vi "Alter Macro V2.vi"(7 "Action":enum16{"Add", "Insert", "Modify", "Delete"}(ring)=enum."Delete", 9 "Step":i32, 10 "Steps in":T1[](array[typedef])) -> (2 "Steps out":T1[](array[typedef]))   [LabVIEW 2023]
doc: "Higher level VI for performing a number of actions on a profile. Takes <B>Action</B> as an input and executes code that performs that action.\n\nThis V2 is meant to be used in conjunction with the double click functionality that was put in as a patch."
uses:
  CTLs/Step Type V3.ctl
  CTLs/Step V3.ctl
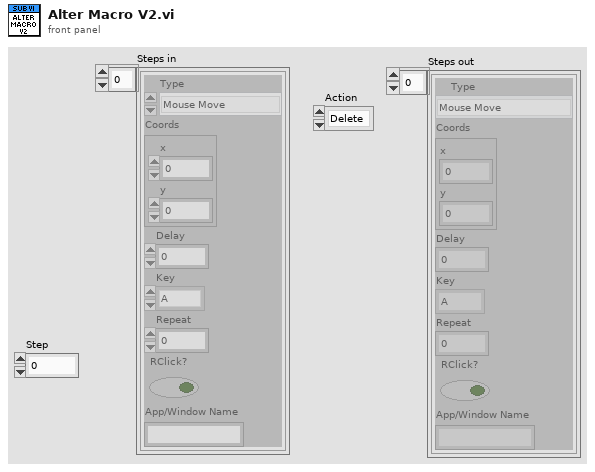
[diagram p1: front panel]
types:
  T1 = typedef "Step V3.ctl" = cluster{"Type":T2, "Coords":cluster{"x":i32, "y":i32}, "Delay":i32, "Key":u8, "Repeat":i32, "RClick?":bool, "App/Window Name":string}
  T2 = typedef "Step Type V3.ctl" = enum16{"Mouse Move", "Mouse Click", "Key Press", "Wait", "Mouse Down", "Mouse Up", "Key Down", "Key Up", "Run Application", "Quit Application", "Maximize Window", "Minimize Window", "Bring Window to Front", "Send Window to Back"}
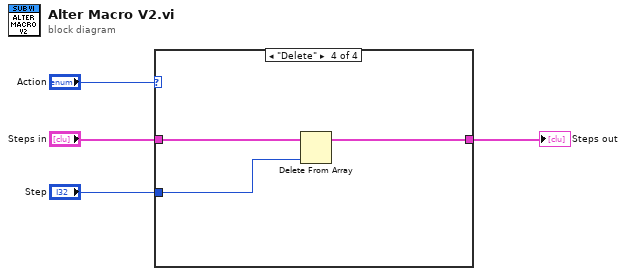
[diagram p0: block diagram]
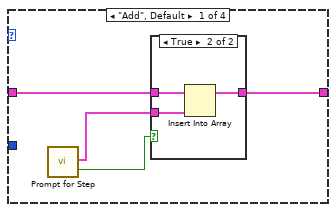
[diagram p2: hidden frame]
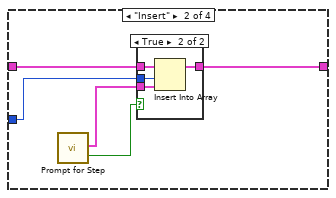
[diagram p4: hidden frame]
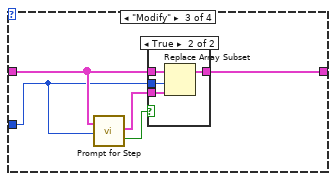
[diagram p6: hidden frame]
diagram:
  n1 = case shown="\"Delete\"" "Action" {
    tunnel: "Steps in" -> [w7 w17 w27 w35]
    tunnel: [w6 w16 w26 w34] -> w1
    tunnel: "Step" -> [_ w13 w23 w33]
    frame "Add", Default {
      n2 = call "Prompt for Step.vi"() -> ("New Data Out"=w8:T1, "OK?"=w5:bool)  [unwired: 17 in, 1 out]
      n3 = case shown="True" w5 {
        tunnel: w8 -> [_ w12]
        tunnel: w7 -> [w9 w11]
        tunnel: [w9 w10] -> w6
        frame False {
        }
        frame True {
          n4 = Insert Into Array(array=w11, new element=w12) -> (w10:T1[])  [unwired: 1 in]
        }
      }
    }
    frame "Insert" {
      n5 = call "Prompt for Step.vi"() -> ("New Data Out"=w15:T1, "OK?"=w14:bool)  [unwired: 17 in, 1 out]
      n6 = case shown="True" w14 {
        tunnel: w13 -> [_ w22]
        tunnel: w15 -> [_ w21]
        tunnel: w17 -> [w18 w20]
        tunnel: [w18 w19] -> w16
        frame False {
        }
        frame True {
          n7 = Insert Into Array(array=w20, index=w22, new element=w21) -> (w19:T1[])
        }
      }
    }
    frame "Modify" {
      n8 = call "Prompt for Step.vi"("Steps"=w27, "Index"=w23) -> ("New Data Out"=w25:T1, "OK?"=w24:bool)  [unwired: 15 in, 1 out]
      n9 = case shown="True" w24 {
        tunnel: w23 -> [_ w32]
        tunnel: w25 -> [_ w31]
        tunnel: [w28 w30] -> w26
        tunnel: w27 -> [w28 w29]
        frame False {
        }
        frame True {
          n10 = Replace Array Subset(array=w29, new element=w31, index=w32) -> (w30:T1[])
        }
      }
    }
    frame "Delete" {
      n11 = Delete From Array(array=w35, index=w33) -> (array with subset deleted=w34:T1[])  [unwired: 1 in, 1 out]
    }
  }
  "Steps out" <- w1
